vi "Extract Lines on Grass (LPF).vi"(6 "error in":errorcluster, 9 "Image In":T1) -> (0 "error out":errorcluster, 3 "Image Out":T1, 5 "Number of Particles":i32)   [LabVIEW 2009]
uses:
  <vilib>/vision/Image Controls.llb/IMAQ Image.ctl
  <vilib>/vision/NI_Vision_Development_Module.lvlib
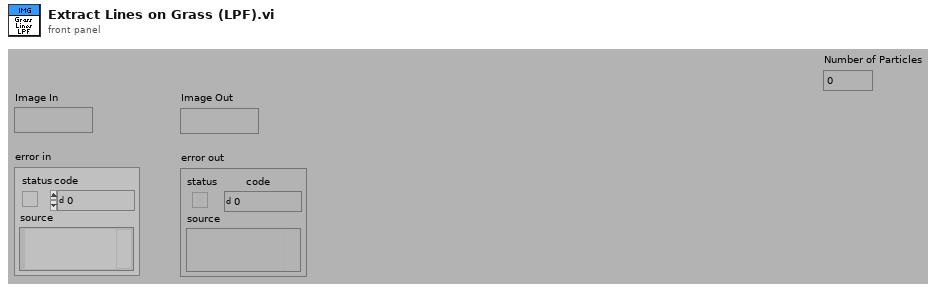
[diagram p1: front panel]
types:
  T1 = typedef "IMAQ Image.ctl" = refnum<image>
  T2 = typedef "Image Type" = u32
  T3 = cluster{"Measurement Parameter":i32, "Range Lower Value":dbl, "Range Upper Value":dbl, "Range":bool, "Measurement Type":bool}[]
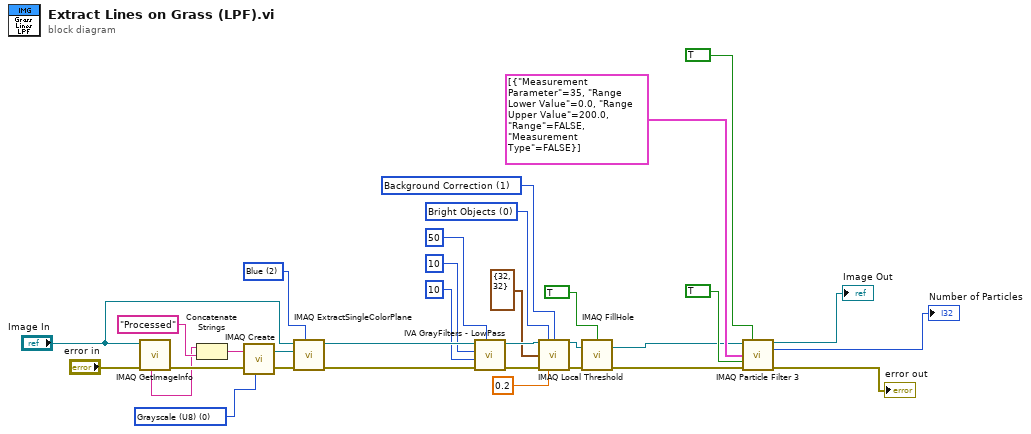
[diagram p0: block diagram]
diagram:
  w11 = T2 0 items=["Grayscale (U8)", "Grayscale (I16)", "Grayscale (SGL)", "Complex (CSG)", "RGB (U32)", "HSL (U32)", "RGB (U64)"] ("Image Type")
  w21 = u32 0 items=["Bright Objects", "Dark Objects"] ("Look For (Bright Objects)")
  w24 = u32 1 items=["Niblack", "Background Correction"] ("Method")
  w32 = 2 items=["Red", "Green", "Blue", "Hue", "Saturation", "Luminance", "Value", "Intensity"] ("Color Plane")
  n1 = call "IMAQ GetImageInfo"("error in (no error)"="error in", "Image"="Image In") -> ("error out"=w10:errorcluster, "Image Name"=w7:string)  [unwired: 8 out]
  n2 = Concatenate Strings(w7, "Processed" ("Image Name")) -> (w8:string)
  n3 = call "IMAQ Create"("Image Name"=w8, "Image Type"=w11, "error in (no error)"=w10) -> ("New Image"=w3:T1, "error out"=w5:errorcluster)  [unwired: 1 in, 1 out]
  n4 = call "IMAQ ExtractSingleColorPlane"("Color Plane"=w32, "error in (no error)"=w5, "Image Dst"=w3, "Image Src"="Image In") -> ("error out"=w31:errorcluster, "Image Dst Out"=w30:T1)  [unwired: 6 out]
  n5 = call <vilib>:"IVA GrayFilters - LowPass.vi"("Tolerance"=50, "error in"=w31, "Filter size Y"=10, "Filter size X"=10, "Image In"=w30) -> ("error out"=w29:errorcluster, "Image Out"=w25:T1)  [unwired: 5 out]
  n6 = call "IMAQ Local Threshold"("Image Src"=w25, "Look For (Bright Objects)"=w21, "Method (Niblack)"=w24, "Window Size (32x32)"=cluster{"SizeX":i32, "SizeY":i32} {"SizeX"=32, "SizeY"=32} ("Kernel Size"), "error in (no error)"=w29, "Niblack Deviation Factor (0.2)"=0.2 ("Niblack Deviation Factor")) -> ("Image Dst Out"=w18:T1, "error out"=w20:errorcluster)  [unwired: 2 in, 6 out]
  n7 = call "IMAQ FillHole"("error in (no error)"=w20, "Image Src"=w18, "Connectivity 4/8 (8)"=TRUE) -> ("error out"=w1:errorcluster, "Image Dst Out"=w2:T1)  [unwired: 1 in, 2 out]
  n8 = call "IMAQ Particle Filter 3"("Image Src"=w2, "Connectivity 4/8 (8)"=TRUE, "Selection Values"=T3 [{"Measurement Parameter"=35, "Range Lower Value"=0.0, "Range Upper Value"=200.0, "Range"=FALSE, "Measurement Type"=FALSE}], "Keep/Remove Particles (F)"=TRUE ("Keep/Remove Particles"), "error in (no error)"=w1) -> ("Image Dst Out"=→"Image Out":T1, "Number of Particles"=→"Number of Particles":i32, "error out"=→"error out":errorcluster)  [unwired: 4 in, 4 out]
